vi "Measure Capacitance at Marker.vi"(0 "VISA resource name":refnum<visa-resource-name>="E5080A", 2 "Meas Type":T2, 5 "Averaging Count":i32=3, 11 "Error In":errorcluster) -> (4 "Marker Measurements":T1 {"Port 3 Capacitance" format="%#_6p"; "Port 2 Capacitance" format="%#_6p"; "Port 1 Capacitance" format="%#_6p"}, 15 "Error Out":errorcluster)   [LabVIEW 2013]
uses:
  Controls/Meas Type.ctl
  Controls/ENA_Marker Measurements.ctl
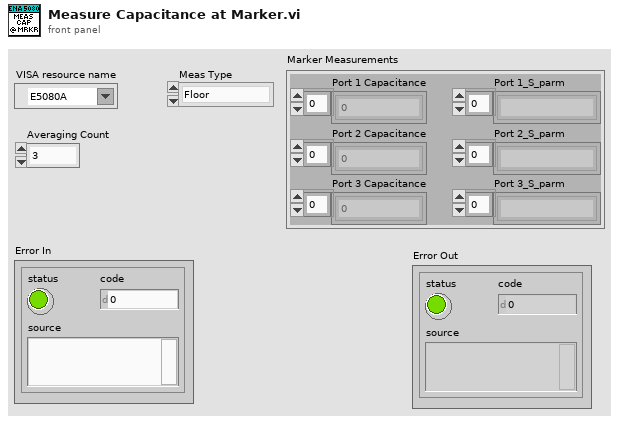
[diagram p1: front panel]
types:
  T1 = typedef "ENA_Marker Measurements.ctl" = cluster{"Port 1 Capacitance":dbl[], "Port 2 Capacitance":dbl[], "Port 3 Capacitance":dbl[], "Port 1_S_parm":string[], "Port 2_S_parm":string[], "Port 3_S_parm":string[]}
  T2 = typedef "Meas Type.ctl" = enum16{"Floor", "Roof", "Buckling", "Charge Transfer"}
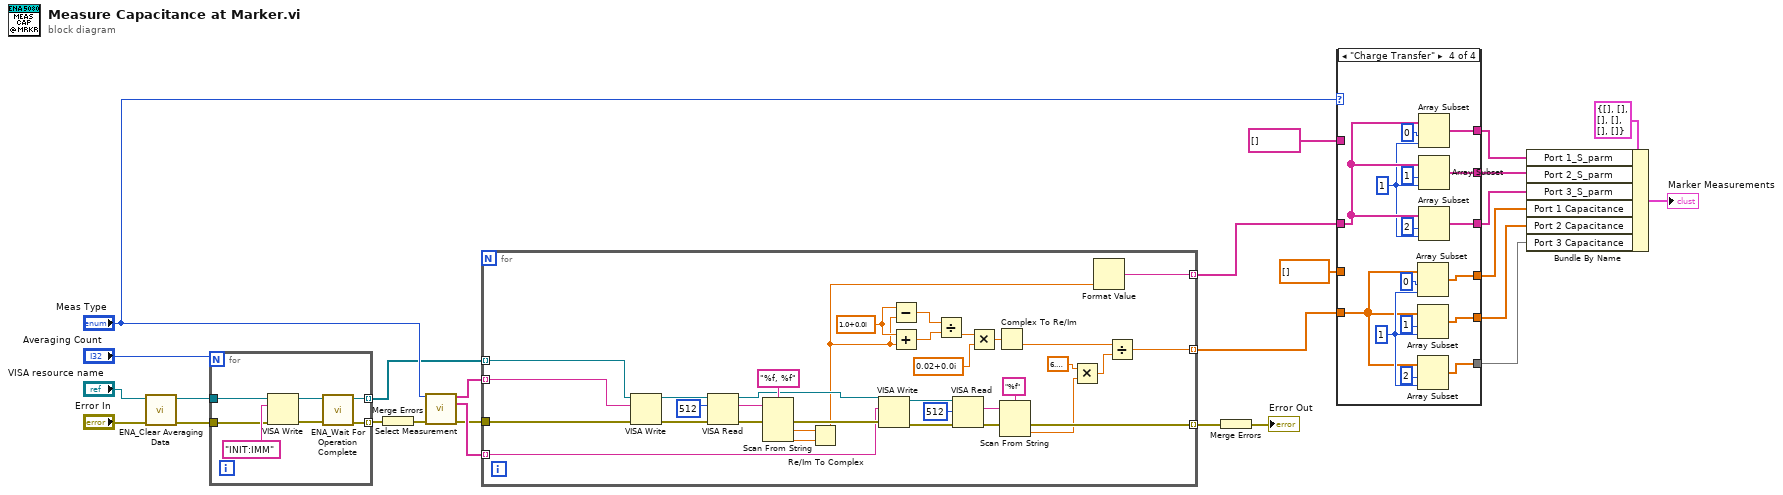
[diagram p0: block diagram]
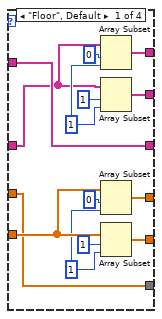
[diagram p2: hidden frame]
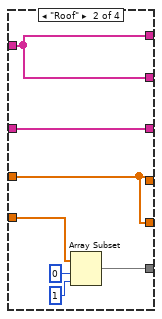
[diagram p3: hidden frame]
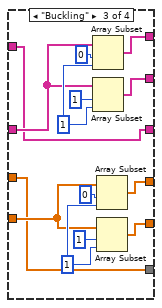
[diagram p4: hidden frame]
diagram:
  n1 = call "ENA_Clear Averaging Data.vi"("error in (no error)"="Error In", "VISA resource name"="VISA resource name") -> ("error out"=w17:errorcluster, "VISA resource name out"=w16:refnum<visa-resource-name>)  [unwired: 8 in]
  n2 = for {
    N: "Averaging Count" -> [_]
    tunnel: w17 -> [w32]
    tunnel: w16 -> [w31]
    tunnel: [w28] -> w14 mode=indexing
    tunnel: [w27] -> w13 mode=indexing
    n3 = VISA Write(VISA resource name=w31, write buffer="INIT:IMM" ("format string"), error in (no error)=w32) -> (VISA resource name out=w29:refnum<visa-resource-name>, error out=w30:errorcluster)  [unwired: 1 out]
    n4 = call "ENA_Wait For Operation Complete.vi"("error in (no error)"=w30, "VISA resource name"=w29) -> ("error out"=w27:errorcluster, "VISA resource name out"=w28:refnum<visa-resource-name>)  [unwired: 8 in]
  }
  n5 = Merge Errors(w13) -> (w12:errorcluster)
  n6 = call "Select Measurement.vi"("Meas Type"="Meas Type", "Error In"=w12) -> ("Y axis commands>>>"=w26:string[], "X axix commands>>>"=w25:string[], "Error Out"=w24:errorcluster)  [unwired: 11 in]
  n7 = for {
    tunnel: w26 -> [w60] mode=indexing
    tunnel: w25 -> [w52] mode=indexing
    tunnel: w14 -> [w61] mode=indexing
    tunnel: w24 -> [w50]
    tunnel: [w49] -> w23 mode=indexing
    tunnel: [w36] -> w20 mode=indexing
    tunnel: [w34] -> w10 mode=indexing
    w42 = cdb 1.0+0.0i
    n8 = VISA Write(VISA resource name=w61, write buffer=w60, error in (no error)=w50) -> (VISA resource name out=w66:refnum<visa-resource-name>, error out=w67:errorcluster)  [unwired: 1 out]
    n9 = VISA Read(VISA resource name=w66, byte count=u32 512, error in (no error)=w67) -> (VISA resource name out=w51:refnum<visa-resource-name>, read buffer=w64:string, error out=w62:errorcluster)  [unwired: 1 out]
    n10 = Scan From String(format string="%f, %f", input string=w64, error in=w62) -> (error out=w53:errorcluster, output 1=w48:dbl, output 2=w47:dbl)  [unwired: 3 in, 2 out]
    n11 = Re/Im To Complex(1:w47, 2:w48) -> (0:w35:cdb)
    n12 = VISA Write(VISA resource name=w51, write buffer=w52, error in (no error)=w53) -> (VISA resource name out=w58:refnum<visa-resource-name>, error out=w59:errorcluster)  [unwired: 1 out]
    n13 = Subtract(x=w42, y=w35) -> (x-y=w46:cdb)
    n14 = Add(x=w42, y=w35) -> (x+y=w45:cdb)
    n15 = Divide(x=w46, y=w45) -> (x/y=w44:cdb)
    n16 = VISA Read(VISA resource name=w58, byte count=u32 512, error in (no error)=w59) -> (read buffer=w56:string, error out=w54:errorcluster)  [unwired: 2 out]
    n17 = Multiply(x=w44, y=cdb 0.02+0.0i) -> (x*y=w40:cdb)
    n18 = Complex To Re/Im(x + iy=w40) -> (y=w39:dbl)  [unwired: 1 out]
    n19 = Scan From String(format string="%f", input string=w56, error in=w54) -> (error out=w49:errorcluster, output 1=w37:dbl)  [unwired: 2 in, 2 out]
    n20 = Multiply(x=6.283185307179586, y=w37) -> (x*y=w38:dbl)
    n21 = Format Value(value (0)=w35) -> (output string=w34:string)  [unwired: 2 in]
    n22 = Divide(x=w39, y=w38) -> (x/y=w36:dbl)
  }
  n23 = Merge Errors(w23) -> (→"Error Out":errorcluster)
  n24 = case shown="\"Charge Transfer\"" "Meas Type" {
    tunnel: w20 -> [w78 w87 w94 w106]
    tunnel: [w80 w85 w90 w105] -> w6
    tunnel: [w77 w85 w89 w104] -> w5
    tunnel: [w76 w86 w93 w103] -> w4
    tunnel: dbl[] [] -> [w76 w85 w93 _]
    tunnel: w10 -> [w68 w83 w99 w114]
    tunnel: [w74 w83 w98 w111] -> w1
    tunnel: string[] [] ("Port 1 S-parm") -> [w74 w82 w98 _]
    tunnel: [w70 w82 w91 w115] -> w3
    tunnel: [w69 w82 w92 w116] -> w2
    frame "Floor", Default {
      w71 = 1 ("index")
      w75 = 1 ("index")
      n25 = Array Subset(array=w68, index=0, length=w71) -> (w70:string[])
      n26 = Array Subset(array=w68, index=1, length=w71) -> (w69:string[])
      n27 = Array Subset(array=w78, index=0, length=w75) -> (w80:dbl[])
      n28 = Array Subset(array=w78, index=1, length=w75) -> (w77:dbl[])
    }
    frame "Roof" {
      n29 = Array Subset(array=w87, index=0, length=1 ("index")) -> (w86:dbl[])
    }
    frame "Buckling" {
      w95 = 1 ("index")
      w100 = 1 ("index")
      n30 = Array Subset(array=w99, index=0, length=w100) -> (w91:string[])
      n31 = Array Subset(array=w99, index=1, length=w100) -> (w92:string[])
      n32 = Array Subset(array=w94, index=0, length=w95) -> (w90:dbl[])
      n33 = Array Subset(array=w94, index=1, length=w95) -> (w89:dbl[])
    }
    frame "Charge Transfer" {
      w107 = 1 ("index")
      w112 = 1 ("index")
      n34 = Array Subset(array=w106, index=0, length=w107) -> (w105:dbl[])
      n35 = Array Subset(array=w106, index=1, length=w107) -> (w104:dbl[])
      n36 = Array Subset(array=w106, index=2, length=w107) -> (w103:dbl[])
      n37 = Array Subset(array=w114, index=0, length=w112) -> (w115:string[])
      n38 = Array Subset(array=w114, index=1, length=w112) -> (w116:string[])
      n39 = Array Subset(array=w114, index=2, length=w112) -> (w111:string[])
    }
  }
  n40 = Bundle By Name(cluster=T1 {"Port 1 Capacitance"=[], "Port 2 Capacitance"=[], "Port 3 Capacitance"=[], "Port 1_S_parm"=[], "Port 2_S_parm"=[], "Port 3_S_parm"=[]} ("Marker Measurements 2"), "Port 1_S_parm"=w3, "Port 2_S_parm"=w2, "Port 3_S_parm"=w1, "Port 1 Capacitance"=w6, "Port 2 Capacitance"=w5, "Port 3 Capacitance"=w4) -> (→"Marker Measurements":T1)
